vi "TestExec.Configure Reports, Parse CSV File Row.vi"(11 "Array":string[](array[string])) -> (3 "Report Config Item":T1)   [LabVIEW 2018]
uses:
  Reports/Report.Report File Config Item.ctl
  Reports/Report.Report File Type.ctl
  <vilib>/KATE/Files/File Utils.lvlib
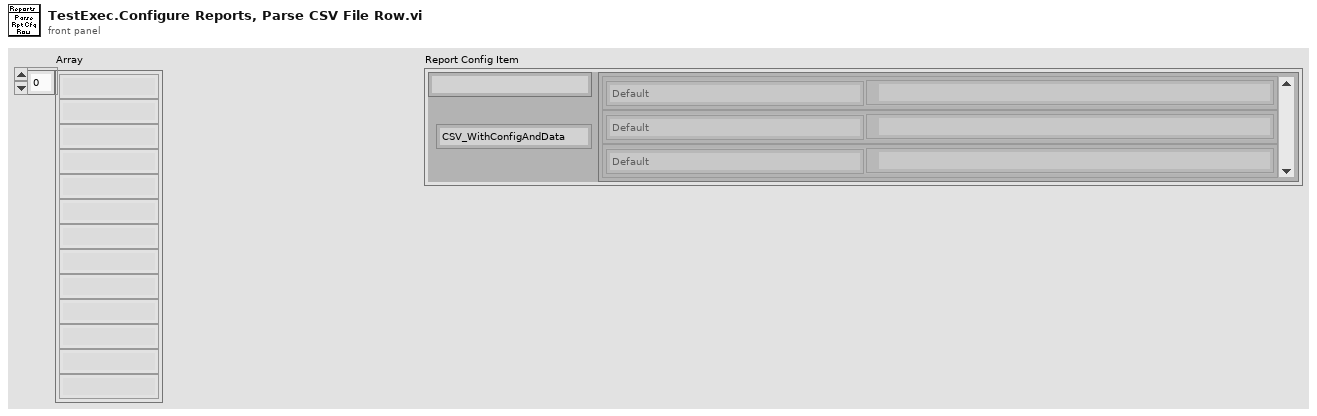
[diagram p1: front panel]
types:
  T1 = typedef "Report.Report File Config Item.ctl" = cluster{"Name":string, "Type":T2, "Seq_Dir":cluster{"Sequence":string, "Folder":path}[]}
  T2 = typedef "Report.Report File Type.ctl" = enum16{"CSV_WithConfigAndData", "CSV", "CSV_SummaryResult", "JSON", "JSON_WithFiles", "XLINK", "XLINK_ResultOnly", "SFC1", ""}
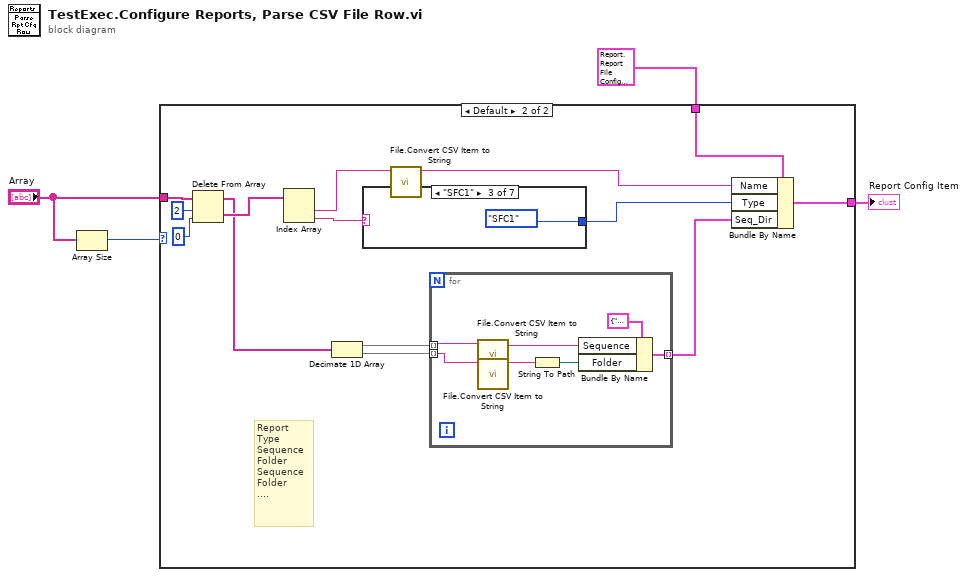
[diagram p0: block diagram]
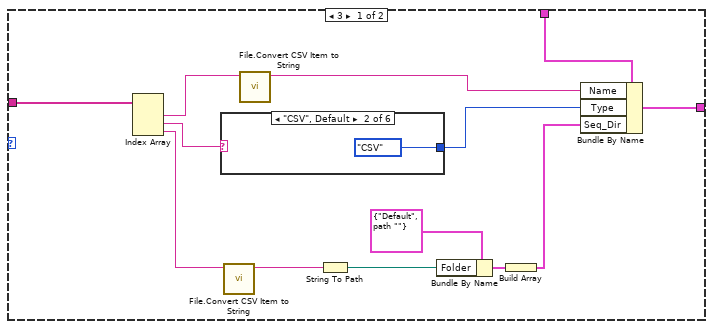
[diagram p2: hidden frame]
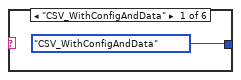
[diagram p3: hidden frame]
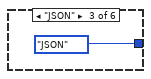
[diagram p4: hidden frame]
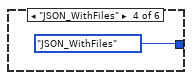
[diagram p5: hidden frame]
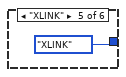
[diagram p6: hidden frame]
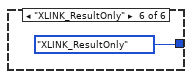
[diagram p7: hidden frame]
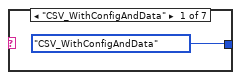
[diagram p8: hidden frame]
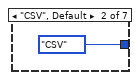
[diagram p9: hidden frame]
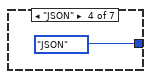
[diagram p10: hidden frame]
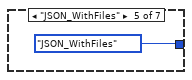
[diagram p11: hidden frame]
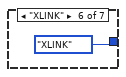
[diagram p12: hidden frame]
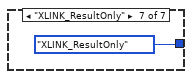
[diagram p13: hidden frame]
diagram:
  n1 = Array Size(array="Array") -> (size(s)=w2:i32)
  n2 = case shown="Default" w2 {
    tunnel: T1 {"Name"="", "Type"=enum."CSV_WithConfigAndData", "Seq_Dir"=[]} ("Report Config Item") -> [w17 w37]
    tunnel: [w10 w32] -> w3
    tunnel: "Array" -> [w9 w31]
    frame 3 {
      n3 = Index Array(array=w9) -> (element #1=w12:string, element #2=w16:string, element #3=w14:string)  [unwired: 3 in]
      n4 = case shown="\"CSV\", Default" w16 {
        tunnel: [Report.Report_File_Type."CSV_WithConfigAndData" ("Type") Report.Report_File_Type."CSV" ("Type") Report.Report_File_Type."JSON" ("Type") Report.Report_File_Type."JSON_WithFiles" ("Type") Report.Report_File_Type."XLINK" ("Type") Report.Report_File_Type."XLINK_ResultOnly" ("Type")] -> w15
        frame "CSV_WithConfigAndData" {
        }
        frame "CSV", Default {
        }
        frame "JSON" {
        }
        frame "JSON_WithFiles" {
        }
        frame "XLINK" {
        }
        frame "XLINK_ResultOnly" {
        }
      }
      n5 = call <vilib>:"File.Convert CSV Item to String.vi"("String"=w14) -> ("String Out"=w13:string)  [unwired: 10 in]
      n6 = call <vilib>:"File.Convert CSV Item to String.vi"("String"=w12) -> ("String Out"=w11:string)  [unwired: 10 in]
      n7 = String To Path(string=w13) -> (path=w7:path)
      n8 = Bundle By Name(cluster=cluster{"Sequence":string, "Folder":path} {"Sequence"="Default", "Folder"=path ""} ("Cluster"), "Folder"=w7) -> (w6:cluster{"Sequence":string, "Folder":path})
      n9 = Build Array(w6) -> (w5:cluster{"Sequence":string, "Folder":path}[])
      n10 = Bundle By Name(cluster=w17, "Name"=w11, "Type"=w15, "Seq_Dir"=w5) -> (w10:T1)
    }
    frame Default {
      # "Report\nType\nSequence\nFolder\nSequence\nFolder\n...."
      n11 = Delete From Array(array=w31, length=2, index=0) -> (deleted portion=w28:string[], array with subset deleted=w27:string[])
      n12 = Index Array(array=w28) -> (element #1=w34:string, element #2=w36:string)  [unwired: 2 in]
      n13 = Decimate 1D Array(w27) -> (w26:string[], w25:string[])
      n14 = case shown="\"SFC1\"" w36 {
        tunnel: [Report.Report_File_Type."CSV_WithConfigAndData" ("Type") Report.Report_File_Type."CSV" ("Type") Report.Report_File_Type."SFC1" ("Type") Report.Report_File_Type."JSON" ("Type") Report.Report_File_Type."JSON_WithFiles" ("Type") Report.Report_File_Type."XLINK" ("Type") Report.Report_File_Type."XLINK_ResultOnly" ("Type")] -> w35
        frame "CSV_WithConfigAndData" {
        }
        frame "CSV", Default {
        }
        frame "SFC1" {
        }
        frame "JSON" {
        }
        frame "JSON_WithFiles" {
        }
        frame "XLINK" {
        }
        frame "XLINK_ResultOnly" {
        }
      }
      n15 = call <vilib>:"File.Convert CSV Item to String.vi"("String"=w34) -> ("String Out"=w33:string)  [unwired: 10 in]
      n16 = for {
        tunnel: w26 -> [w40] mode=indexing
        tunnel: w25 -> [w39] mode=indexing
        tunnel: [w38] -> w24 mode=indexing
        n17 = call <vilib>:"File.Convert CSV Item to String.vi"("String"=w40) -> ("String Out"=w41:string)  [unwired: 10 in]
        n18 = call <vilib>:"File.Convert CSV Item to String.vi"("String"=w39) -> ("String Out"=w44:string)  [unwired: 10 in]
        n19 = String To Path(string=w44) -> (path=w42:path)
        n20 = Bundle By Name(cluster=cluster{"Sequence":string, "Folder":path} {"Sequence"="Default", "Folder"=path ""} ("Cluster"), "Sequence"=w41, "Folder"=w42) -> (w38:cluster{"Sequence":string, "Folder":path})
      }
      n21 = Bundle By Name(cluster=w37, "Name"=w33, "Type"=w35, "Seq_Dir"=w24) -> (w32:T1)
    }
  }
  "Report Config Item" <- w3
